vi "SubVI_TIPS.vi"() -> ()   [LabVIEW 2014]
panel:
  in  "Enter":bool
  # "遊戲規則：\n \n             1. 遊戲中共有五題，由系統隨機出題，並要求玩家需\n                 於指定時限內依序輸入各電阻顏色所對應之電阻值\n\n             2. 若所輸入之數值與其電阻值不符，則必須重新答題\n                 其中，若累積輸入三次錯誤，則遊戲立即結束！！\n                 在五題皆回答正確後，記錄所花費之時間於英雄榜\n                 上並進行排名比較\n\n尬電小技巧：\n \n             1. 在按下 START 按鈕後，可利用 Tab 與 Enter 鍵快\n                 速切換數值欄位與答題按鈕\n\n             2. 電阻顏色與所對應之數值 可按下 HELP 按鈕查詢"
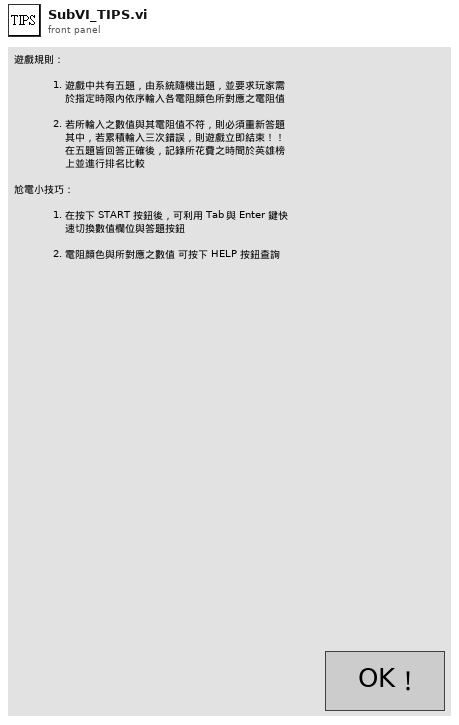
[diagram p1: front panel]
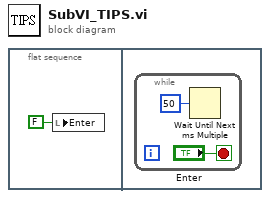
[diagram p0: block diagram]
diagram:
  n1 = flat-sequence {
    frame #0 {
      n2 = local write "Enter"(FALSE ("Enter")) -> ()
    }
    frame #1 {
      n3 = while {
        stop <- "Enter" stop-if-true
        n4 = Wait Until Next ms Multiple(millisecond multiple=u32 50 ("milliseconds to wait")) -> ()  [unwired: 1 out]
      }
    }
  }
